vi "StepsTableToStepsArray.vi"(4 "Steps Table Input":string[][](table)) -> (1 "Steps Array Output":T1[](array[typedef]) {"Duration" min=0.0 max=100.0 format="%.2f"; "Fire" min=0.0 max=100.0 format="%.2f %"})   [LabVIEW 2024]
uses:
  Support/Step.ctl
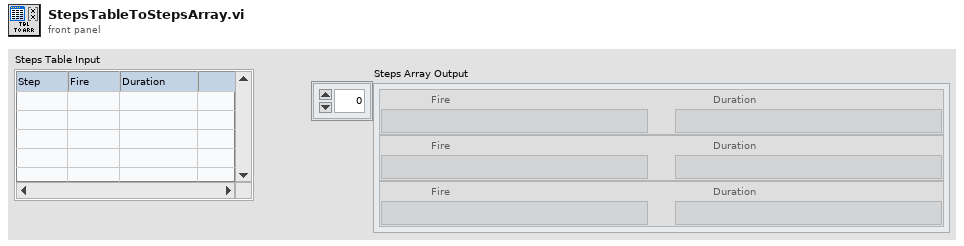
[diagram p1: front panel]
types:
  T1 = typedef "Step.ctl" = cluster{"Fire":dbl, "Duration":dbl}
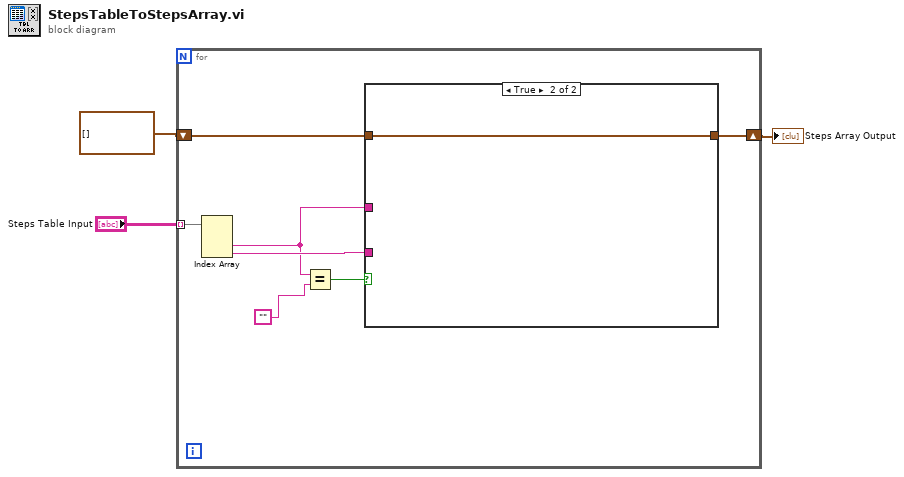
[diagram p0: block diagram]
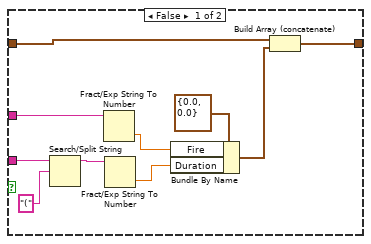
[diagram p2: hidden frame]
diagram:
  n1 = for {
    tunnel: "Steps Table Input" -> [w7] mode=indexing
    shift-right: [w5] -> w2
    shift-left: T1[] [] -> [w4]
    n2 = Index Array(array=w7) -> (element #2=w9:string, element #3=w10:string)  [unwired: 3 in, 1 out]
    n3 = Equal?(x=w9, y="") -> (x = y?=w6:bool)
    n4 = case shown="True" w6 {
      tunnel: w10 -> [w15 _]
      tunnel: w9 -> [w14 _]
      tunnel: [w12 w21] -> w5
      tunnel: w4 -> [w11 w21]
      frame False {
        n5 = Search/Split String(string=w15, search string/char (-)="(") -> (substring before match=w16:string)  [unwired: 1 in, 2 out]
        n6 = Fract/Exp String To Number(string=w14) -> (number=w19:dbl)  [unwired: 3 in, 1 out]
        n7 = Fract/Exp String To Number(string=w16) -> (number=w18:dbl)  [unwired: 3 in, 1 out]
        n8 = Bundle By Name(cluster=T1 {"Fire"=0.0, "Duration"=0.0} ("Step"), "Fire"=w19, "Duration"=w18) -> (w13:T1)
        n9 = Build Array (concatenate)(w11, w13) -> (w12:T1[])
      }
      frame True {
      }
    }
  }
  "Steps Array Output" <- w2
